vi "dcs_rtl_vis.vi"() -> ()   [LabVIEW 2020]
uses:
  <vilib>/Utility/file.llb/Read Delimited Spreadsheet (DBL).vi
panel:
  out "size(s) 2":i32
  in  "milliseconds to wait":u32
  out "Waveform Graph 3":dbl[][](graph)
  out "size(s) 4":i32[](array[numeric])
  out "Numeric":i32
  out "concatenated string":string
  out "size(s)":i32
  out "filenames":string[](array[string])
  in  "file path (dialog if empty) 2":path
  out "all rows 2":dbl[][](array[numeric])
  out "Waveform Graph 2":dbl[][](graph)
  out "Waveform Graph":dbl[][](graph)
  out "all rows":dbl[][](array[numeric])
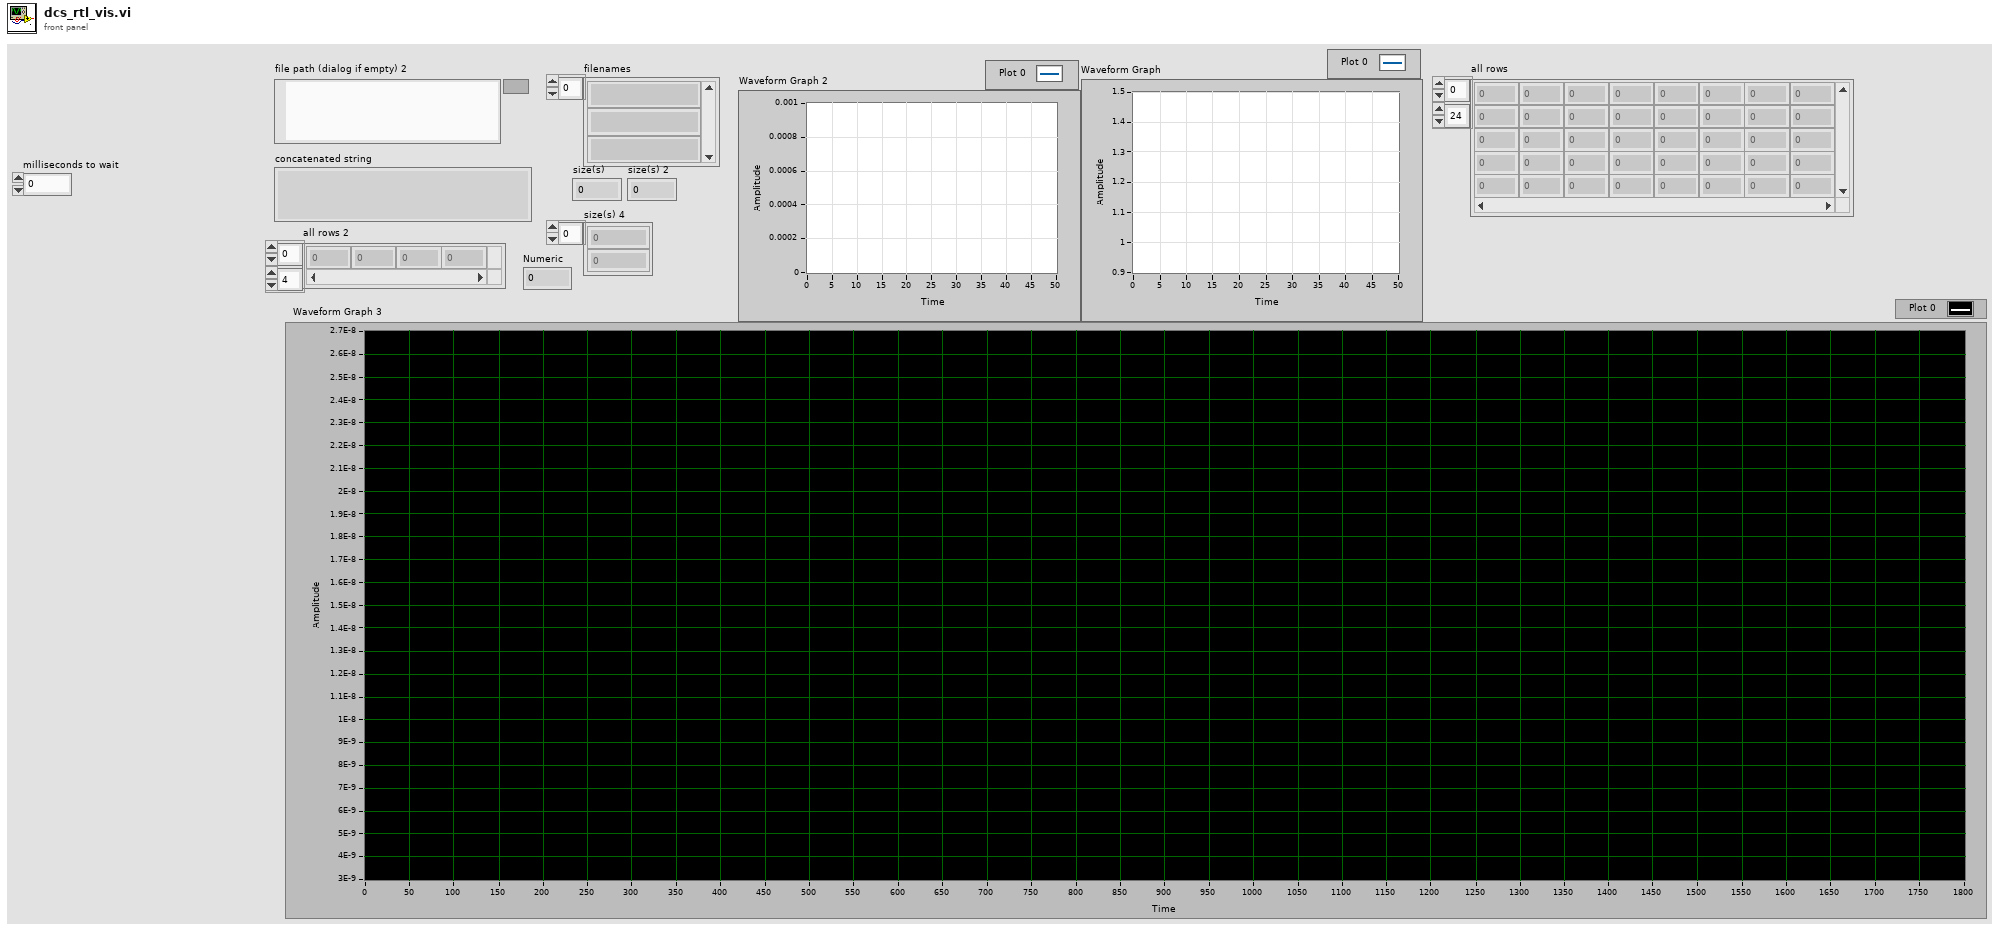
[diagram p1: front panel]
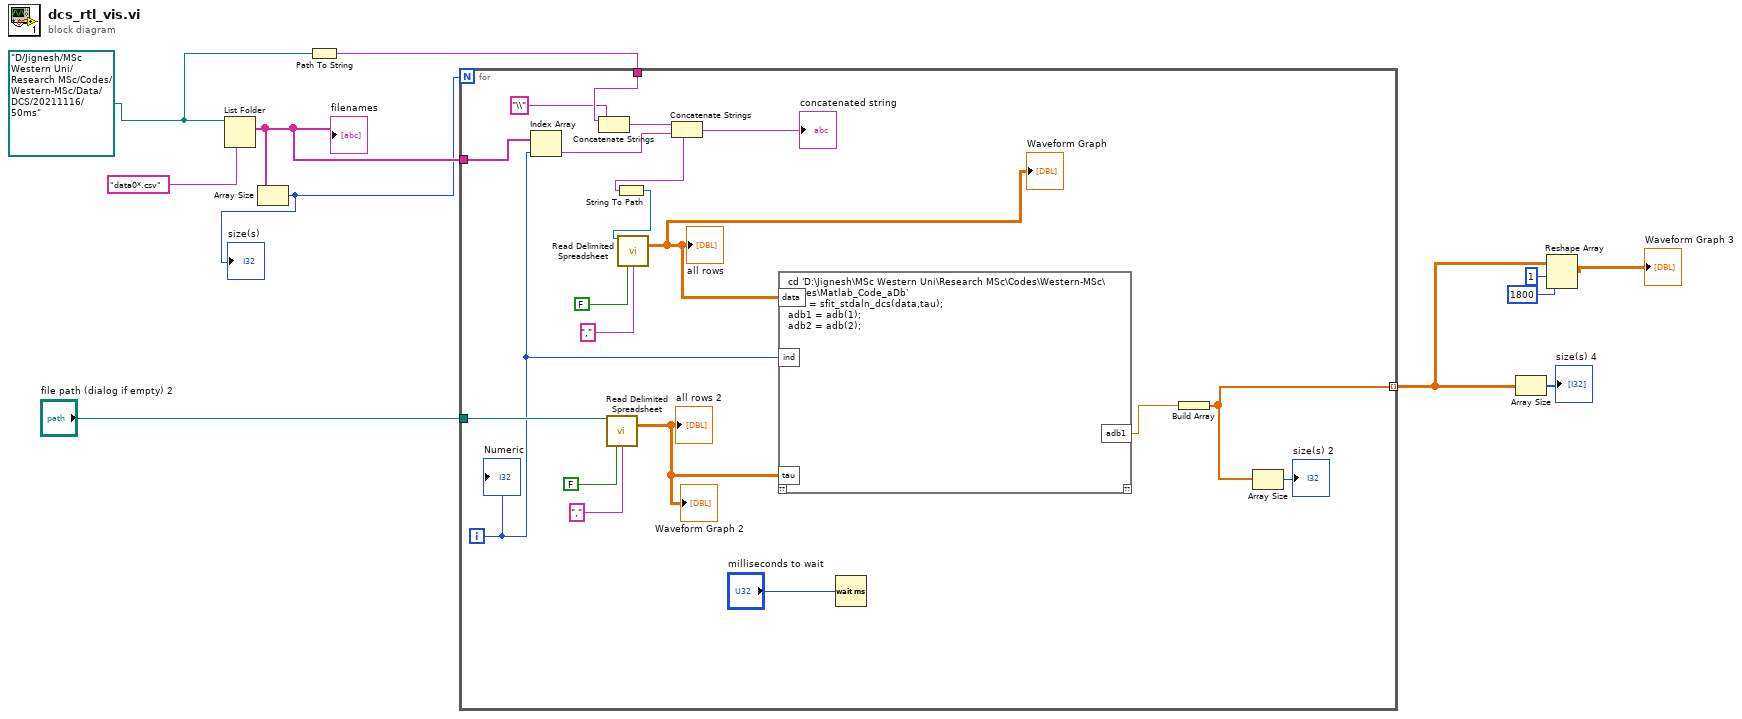
[diagram p0: block diagram]
diagram:
  w8 = path "D:/Jignesh/MSc Western Uni/Research MSc/Codes/Western-MSc/Data/DCS/20211116/50ms"
  n1 = List Folder(path=w8, pattern="data0*.csv") -> (filenames=w10:string[])  [unwired: 2 in, 3 out]
  "filenames" <- w10
  n2 = Array Size(array=w10) -> (size(s)=w7:i32)
  "size(s)" <- w7
  n3 = Path To String(path=w8) -> (string=w9:string)
  n4 = for {
    N: w7 -> [_]
    tunnel: "file path (dialog if empty) 2" -> [w26]
    tunnel: w10 -> [w23]
    tunnel: w9 -> [w19]
    tunnel: [w17] -> w5 mode=indexing
    i -> [w12]
    n5 = Index Array(array=w23, index=w12) -> (element=w22:string)
    n6 = Concatenate Strings(w19, "\\" ("string")) -> (w18:string)
    n7 = call-poly <vilib>:"Read Delimited Spreadsheet.vi"("file path (dialog if empty)"=w26, "transpose? (F)"=FALSE, "delimiter (\\t)"="," ("delimiter (\\t)")) -> ("all rows"=w25:dbl[][])  [unwired: 7 in, 5 out]
    "all rows 2" <- w25
    "Waveform Graph 2" <- w25
    n8 = Concatenate Strings(w18, w22) -> (w21:string)
    "concatenated string" <- w21
    n9 = String To Path(string=w21) -> (path=w20:path)
    n10 = call-poly <vilib>:"Read Delimited Spreadsheet.vi"("file path (dialog if empty)"=w20, "transpose? (F)"=FALSE, "delimiter (\\t)"="," ("delimiter (\\t)")) -> ("all rows"=w24:dbl[][])  [unwired: 7 in, 5 out]
    "all rows" <- w24
    "Waveform Graph" <- w24
    n11 = script code="cd 'D:\\Jignesh\\MSc Western Uni\\Research MSc\\Codes\\Western-MSc\\Codes\\Matlab_Code_aDb'\nadb = sfit_stdaln_dcs(data,tau);\nadb1 = adb(1);\nadb2 = adb(2);"("data"=w24, "tau"=w25, "ind"=w12) -> ("adb1"=w13:dbl)  [unwired: 1 in, 1 out]
    n12 = Wait (ms)(milliseconds to wait="milliseconds to wait") -> ()  [unwired: 1 out]
    n13 = Build Array(w13) -> (w17:dbl[])
    n14 = Array Size(array=w17) -> (size(s)=→"size(s) 2":i32)
    "Numeric" <- w12
  }
  n15 = Array Size(array=w5) -> (size(s)=→"size(s) 4":i32[])
  n16 = Reshape Array(w5, 1 ("dimension size"), 1800 ("dimension size")) -> (→"Waveform Graph 3":dbl[][])
